vi "Variables.vi"(11 "Sequence Config in":refnum<class "Sequence Config.lvclass">) -> (2 "Variables":map{string, dbl}(c390), 3 "Sequence Config out":refnum<class "Sequence Config.lvclass">)   [LabVIEW 2020, in "VolatusSeqConfig.lvlib" / "Sequence Config.lvclass"]
uses:
  Sequence Config.lvclass
  Sequence Config.lvclass/Sequence Config.ctl
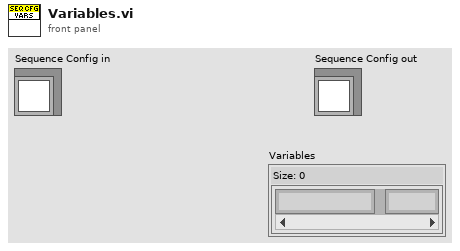
[diagram p1: front panel]
types:
  T1 = typedef "VolatusSeqConfig.lvlib/Variable.ctl" = cluster{"Name":string, "Value":dbl, "Comment":string}
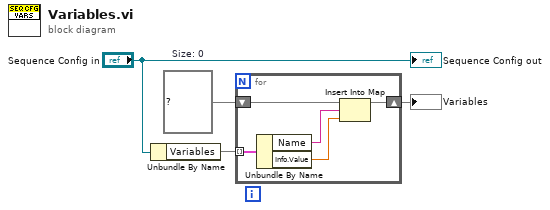
[diagram p0: block diagram]
diagram:
  w2 = map{string, dbl} {}  # Size: 0
  n1 = Unbundle By Name("Sequence Config in") -> ("Variables"=w3:map{string, T1})
  n2 = for {
    tunnel: w3 -> [w9] mode=indexing
    shift-right: [w7] -> w1
    shift-left: w2 -> [w8]
    n3 = Unbundle By Name(w9) -> ("Name"=w6:string, "Info.Value"=w5:dbl)
    n4 = Insert Into Map(map in=w8, key=w6, value=w5) -> (map out=w7:map{string, dbl})  [unwired: 2 out]
  }
  "Variables" <- w1
  "Sequence Config out" <- "Sequence Config in"
